vi "Lab12.vi"() -> ()   [LabVIEW 2022 SP3]
uses:
  <vilib>/DAQmx/read.llb/DAQmx Read (Analog 1D Wfm NChan NSamp).vi
  <vilib>/DAQmx/create/channels.llb/DAQmx Create Channel (AI-Voltage-Basic).vi
  <vilib>/DAQmx/configure/timing.llb/DAQmx Timing (Sample Clock).vi
  <vilib>/DAQmx/miscellaneous.llb/DAQmx Fill In Error Info.vi
panel:
  in  "Base Path":path
  in  "Timing Parameters":T1={"Sample Rate (Hz)"=10000.0, "Total Samles/Channel"=1000} {"Total Samles/Channel" min=1; "Sample Rate (Hz)" min=0.0 max=500000.0}
  in  "Channel Parameters":T2={"DAQmx Device Name"="Dev1", "Channel Low"=0, "Channel High"=2, "Ring"=10.0} {"Ring" items=["+/- 10V"=10.0, "+/- 5V"=5.0, "+/- 1V"=1.0, "+/- 0.2V"=0.2]; "Channel High" min=0 max=7; "Channel Low" min=0 max=7}
  out "Waveform Graph":waveform(dbl)[](graph)
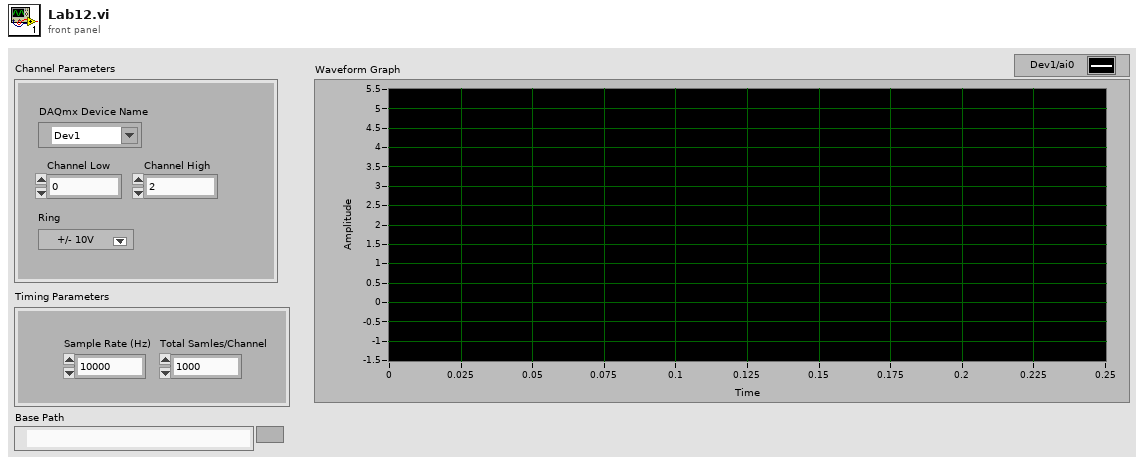
[diagram p1: front panel]
types:
  T1 = cluster{"Sample Rate (Hz)":dbl, "Total Samles/Channel":i32}
  T2 = cluster{"DAQmx Device Name":tag, "Channel Low":i32, "Channel High":i32, "Ring":dbl}
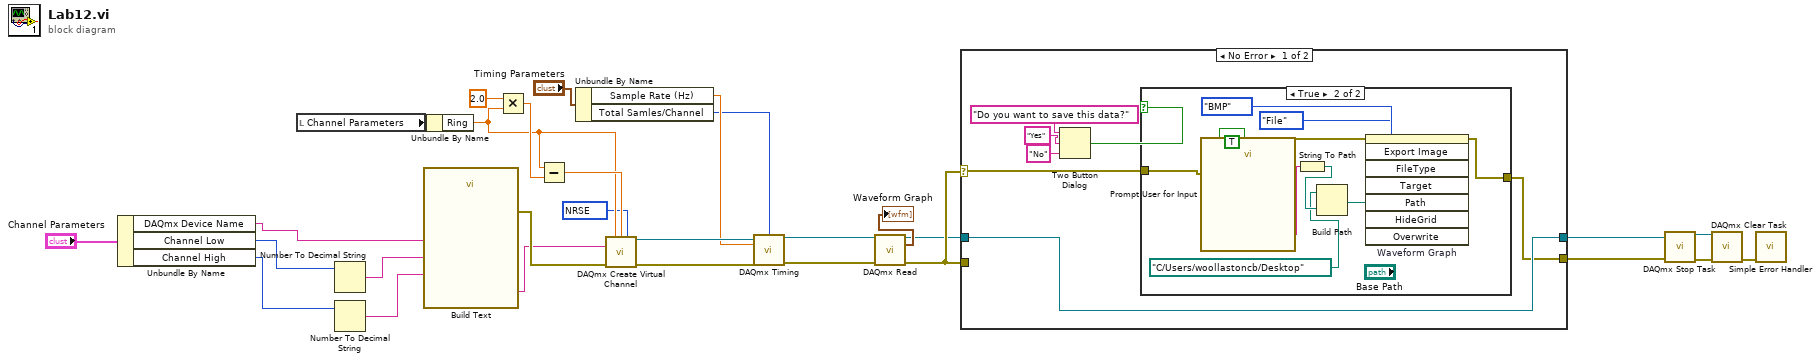
[diagram p0: block diagram]
diagram:
  w1 = 10078 items=["Default"=-1, "RSE"=10083, "NRSE"=10078, "Differential"=10106, "Pseudodifferential"=12529] ("input terminal configuration")
  n1 = Unbundle By Name("Channel Parameters") -> ("DAQmx Device Name"=w13:tag, "Channel Low"=w12:i32, "Channel High"=w11:i32)
  n2 = local read "Channel Parameters"() -> (w10:T2)
  n3 = Number To Decimal String(number=w12) -> (decimal integer string=w29:string)  [unwired: 1 in]
  n4 = Number To Decimal String(number=w11) -> (decimal integer string=w28:string)  [unwired: 1 in]
  n5 = call "Build Text"("Dev"=w13, "lowIn"=w29, "HighIn"=w28) -> ("Result"=w26:string, "error out"=w27:errorcluster)  [unwired: 11 in]
  n6 = Unbundle By Name(w10) -> ("Ring"=w9:dbl)
  n7 = Multiply(x=2.0, y=w9) -> (x*y=w19:dbl)
  n8 = Subtract(x=w9, y=w19) -> (x-y=w18:dbl)
  n9 = Unbundle By Name("Timing Parameters") -> ("Sample Rate (Hz)"=w16:dbl, "Total Samles/Channel"=w15:i32)
  n10 = call-poly <vilib>:"DAQmx Create Virtual Channel.vi"("maximum value"=w9, "minimum value"=w18, "input terminal configuration"=w1, "physical channels"=w26, "error in"=w27) -> ("task out"=w25:refnum<k21>, "error out"=w24:errorcluster)  [unwired: 9 in]
  n11 = call-poly <vilib>:"DAQmx Timing.vi"("task/channels in"=w25, "samples per channel"=w15, "rate"=w16, "error in"=w24) -> ("task out"=w23:refnum<k21>, "error out"=w22:errorcluster)  [unwired: 10 in]
  n12 = call-poly <vilib>:"DAQmx Read.vi"("task/channels in"=w23, "error in"=w22) -> ("task out"=w3:refnum<k21>, "data"=→"Waveform Graph":waveform(dbl)[], "error out"=w5:errorcluster)  [unwired: 11 in]
  n13 = case shown="No Error" w5 {
    tunnel: w5 -> [w32 w49]
    tunnel: [w30 w49] -> w4
    tunnel: [w31 w48] -> w2
    tunnel: w3 -> [w31 w48]
    frame No Error {
      n14 = Two Button Dialog(message="Do you want to save this data?", 1:"No" ("F button name (\"Cancel\")"), 2:"Yes" ("T button name (\"OK\")")) -> (T button?=w36:bool)
      n15 = case shown="True" w36 {
        tunnel: [w37 w45] -> w30
        tunnel: w32 -> [w37 w42]
        frame False {
        }
        frame True {
          n16 = call "Prompt User for Input"("Enable"=TRUE, "error in (no error)"=w42) -> ("File Name"=w41:string, "error out"=w46:errorcluster)  [unwired: 15 in, 1 out]
          n17 = String To Path(string=w41) -> (path=w40:path)
          n18 = Build Path(base path=path "C:/Users/woollastoncb/Desktop", name or relative path=w40) -> (appended path=w38:path)
          n19 = invoke on="Waveform Graph" class="WFGraph (strict)" method="Export Image"(error in=w46, "FileType"=enum32{"BMP", "EPS", "EMF", "PICT"}."BMP" ("File Type"), "Target"=enum32{"File", "Clipboard"}."File", "Path"=w38) -> (error out=w45:errorcluster)  [unwired: 4 in, 7 out]
        }
      }
    }
    frame Error {
    }
  }
  n20 = call <vilib>:"DAQmx Stop Task.vi"("task/channels in"=w2, "error in"=w4) -> ("task out"=w7:refnum<k21>, "error out"=w6:errorcluster)  [unwired: 12 in]
  n21 = call <vilib>:"DAQmx Clear Task.vi"("task in"=w7, "error in"=w6) -> ("error out"=w8:errorcluster)  [unwired: 13 in]
  n22 = call <vilib>:"Simple Error Handler.vi"("error in (no error)"=w8) -> ()  [unwired: 4 in, 5 out]
